vi "Check-Camera-selector.vi"(8 "error in":errorcluster, 10 "Config. params. ref.":refnum<data-value>, 11 "Camera selector":refnum<vi>) -> (0 "error IO":errorcluster)   [LabVIEW 2013, in "CameraVision.lvlib" / "CV-UI.lvclass"]
doc: "This function resets and disables the 'Camera selector' front panel control when only 1 camera is configured."
uses:
  CV-UI.lvclass
  Main/Configuration/CV-Configuration.lvclass
  Main/Configuration/CV-Configuration.lvclass/CV-Configuration.ctl
  Camera-selector.ctl
  Main/Configuration/Read Number of cameras.vi
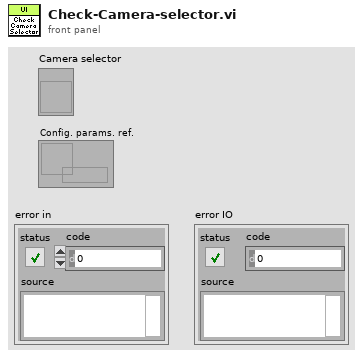
[diagram p1: front panel]
types:
  T1 = typedef "CameraVision.lvlib/CV-UI.lvclass/Camera-selector.ctl" = enum16{"Camera 1", "Camera 2"}
  T2 = enum8{"Enabled", "Disabled", "Disabled and Grayed Out"}
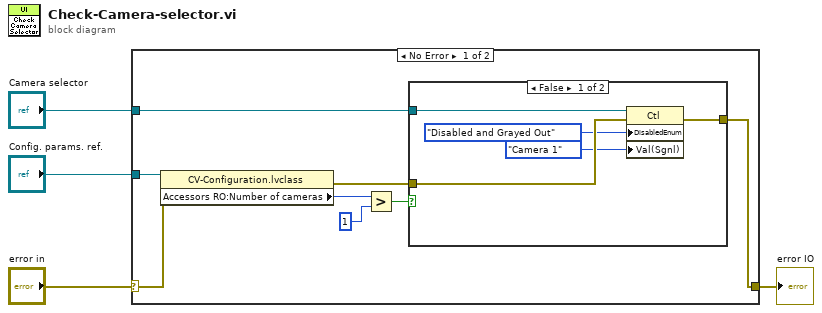
[diagram p0: block diagram]
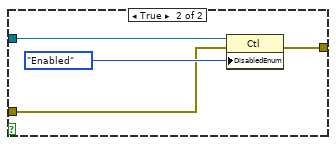
[diagram p2: hidden frame]
diagram:
  n1 = case shown="No Error" "error in" {
    selector: "error in" -> [w8 w22]
    tunnel: "Camera selector" -> [w7 _]
    tunnel: [w5 w22] -> w3
    tunnel: "Config. params. ref." -> [w10 _]
    frame No Error {
      n2 = property class="CV-Configuration.lvclass"(reference=w10, error in=w8) -> (error out=w6:errorcluster, "Accessors RO:Number of cameras"=w9:i32)  [unwired: 1 out]
      n3 = Greater?(x=w9, y=1) -> (0:w11:bool)
      n4 = case shown="False" w11 {
        tunnel: w7 -> [w17 w21]
        tunnel: w6 -> [w15 w19]
        tunnel: [w16 w18] -> w5
        frame False {
          n5 = property class="Ctl"(reference=w17, error in=w15, "DisabledEnum"=T2."Disabled and Grayed Out" ("Disabled"), "Val(Sgnl)"=Camera-selector."Camera 1" ("Value")) -> (error out=w16:errorcluster)  [unwired: 1 out]
        }
        frame True {
          n6 = property class="Ctl"(reference=w21, error in=w19, "DisabledEnum"=T2."Enabled" ("Disabled")) -> (error out=w18:errorcluster)  [unwired: 1 out]
        }
      }
    }
    frame Error {
    }
  }
  "error IO" <- w3
